vi "kalman update step single cycle.vi"(1 "apply measurement?":bool=TRUE, 5 "location":i16, 7 "state in":T2, 9 "num photons":u8, 12 "pixel values cluster":T1) -> (8 "state out":T2)   [LabVIEW 2010]
uses:
  integrating single axis kalman state.ctl
  common_typedefs/channels_cluster.ctl
  <vilib>/rvi/FXPMathLib/FxpSub/XNode/nifxpmath_Sub.xnode
  <vilib>/rvi/FXPMathLib/FxpSub/subVIs/nifxpmath_Sub_SimConfig.ctl
  <vilib>/fxp/LVFixedPointQuantizationPolicyTypeDef.ctl
  <vilib>/fxp/LVFixedPointOverflowPolicyTypeDef.ctl
  <vilib>/rvi/FXPMathLib/FxpMul/XNode/nifxpmath_Multiplier.xnode
  <vilib>/rvi/FXPMathLib/FxpMul/subVIs/nifxpmath_Mul_SimConfig.ctl
  <vilib>/rvi/FXPMathLib/FxpAdd/XNode/nifxpmath_Add.xnode
  <vilib>/rvi/FXPMathLib/FxpAdd/subVIs/nifxpmath_Add_SimConfig.ctl
  <vilib>/rvi/FXPMathLib/FxpSub/simVIs/DllFxpSubTemp_sub.vi
  <vilib>/rvi/FXPMathLib/FxpMul/simVIs/DllFxpMulTemp_sub.vi
  <vilib>/rvi/FXPMathLib/FxpAdd/simVIs/DllFxpAddTemp_sub.vi
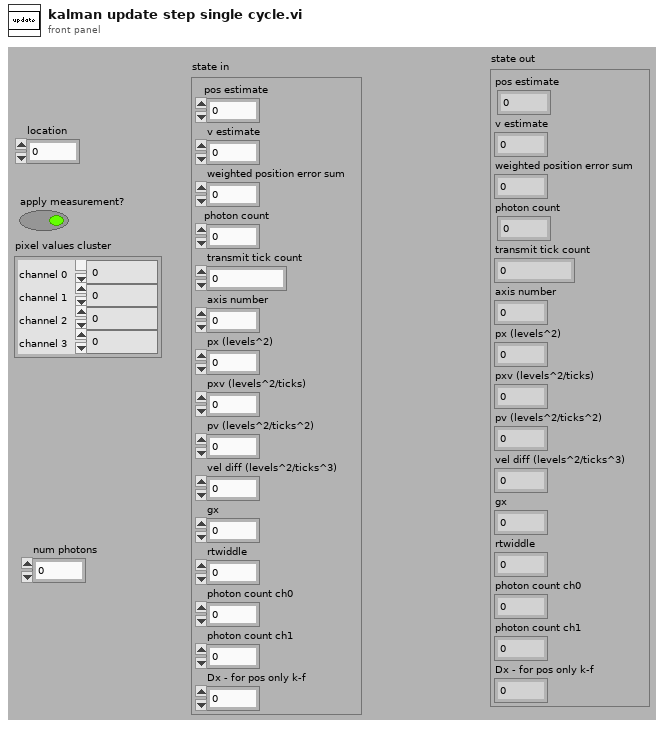
[diagram p1: front panel]
types:
  T1 = typedef "channels_cluster.ctl" = cluster{"channel 0":u32, "channel 1":u32, "channel 2":u32, "channel 3":u32}
  T2 = typedef "integrating single axis kalman state.ctl" = cluster{"pos estimate":fxp<+/-,32,16>, "v estimate":fxp<+/-,16,0>, "weighted position error sum":fxp<+/-,32,32>, "photon count":u32, "transmit tick count":u32, "axis number":u8, "px (levels^2)":fxp<+,32,19>, "pxv (levels^2/ticks)":fxp<+,32,2>, "pv (levels^2/ticks^2)":fxp<+,32,-14>, "vel diff (levels^2/ticks^3)":fxp<+,24,-22>, "gx":fxp<+,16,8>, "rtwiddle":fxp<+,16,26>, "photon count ch0":u32, "photon count ch1":u32, "Dx - for pos only k-f":fxp<+,32,19>}
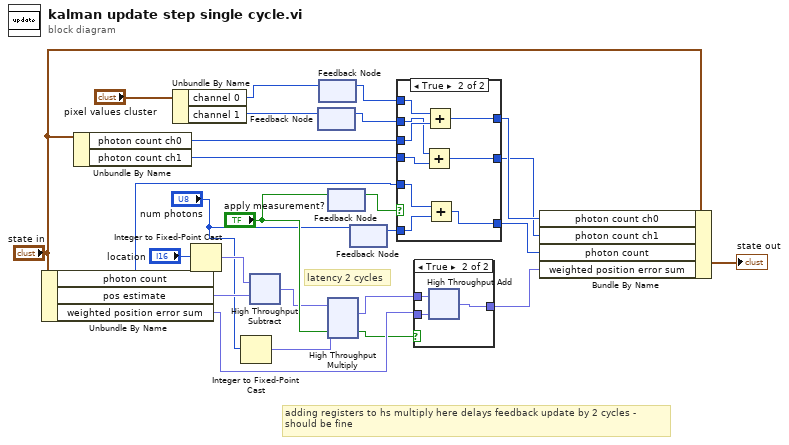
[diagram p0: block diagram]
diagram:
  # "latency 2 cycles"
  # "adding registers to hs multiply here delays feedback update by 2 cycles - \nshould be fine"
  n1 = Unbundle By Name("state in") -> ("photon count"=w18:u32, "pos estimate"=w23:fxp<+/-,32,16>, "weighted position error sum"=w22:fxp<+/-,32,32>)
  n2 = Unbundle By Name("state in") -> ("photon count ch0"=w8:u32, "photon count ch1"=w7:u32)
  n3 = Unbundle By Name("pixel values cluster") -> ("channel 0"=w2:u32, "channel 1"=w1:u32)
  n4 = Integer to Fixed-Point Cast(integer="location") -> (fixed-point=w24:fxp<+/-,16,16>)  [unwired: 1 in]
  n5 = Integer to Fixed-Point Cast(integer="num photons") -> (fixed-point=w14:fxp<+,8,8>)  [unwired: 1 in]
  n6 = xnode "High Throughput Subtract"("x"=w24, "y"=w23) -> ("x-y"=w19:fxp<+/-,16,16>)
  n7 = feedback #1() -> (w5:u32)  [unwired: 1 in]
  n8 = feedback-in #1(w1) -> ()
  n9 = feedback #2() -> (w6:u32)  [unwired: 1 in]
  n10 = feedback-in #2(w2) -> ()
  n11 = feedback-in #3("apply measurement?") -> ()
  n12 = feedback #3() -> (w10:bool)  [unwired: 1 in]
  n13 = xnode "High Throughput Multiply"("x"=w19, "y"=w14, "input valid"="apply measurement?") -> ("x*y"=w13:fxp<+/-,24,24>, "output valid"=w16:bool)  [unwired: 1 in, 1 out]
  n14 = feedback-in #4("num photons") -> ()
  n15 = feedback #4() -> (w12:u8)  [unwired: 1 in]
  n16 = case shown="True" w10 {
    tunnel: w18 -> [w29 w38]
    tunnel: [w29 w36] -> w17
    tunnel: w12 -> [_ w37]
    tunnel: w8 -> [w28 w34]
    tunnel: w7 -> [w27 w32]
    tunnel: w6 -> [_ w35]
    tunnel: w5 -> [_ w33]
    tunnel: [w27 w31] -> w3
    tunnel: [w28 w30] -> w4
    frame False {
    }
    frame True {
      n17 = Add(x=w33, y=w32) -> (x+y=w31:u32)
      n18 = Add(x=w35, y=w34) -> (x+y=w30:u32)
      n19 = Add(x=w38, y=w37) -> (x+y=w36:u32)
    }
  }
  n20 = case shown="True" w16 {
    tunnel: w22 -> [w39 w42]
    tunnel: [w39 w41] -> w21
    tunnel: w13 -> [_ w40]
    frame False {
    }
    frame True {
      n21 = xnode "High Throughput Add"("x"=w40, "y"=w42) -> ("x+y"=w41:fxp<+/-,32,32>)
    }
  }
  n22 = Bundle By Name(cluster="state in", "photon count ch0"=w4, "photon count ch1"=w3, "photon count"=w17, "weighted position error sum"=w21) -> (→"state out":T2)
